vi "Convert RGB to HSV.vi"(11 "Color Box":u32(colorbox)=16777215) -> (1 "V (%)":dbl, 2 "S (%)":dbl, 3 "H (deg)":dbl format="%#_2p")   [LabVIEW 2014, in "HSV Distance Comparison.lvclass"]
doc: "This VI will convert the RGB Color Scale to the HSL Color Scale.\n<b> </b> <b> </b>\n©2017 Q Software Innovations, LLC (QSI)\nwritten by Quentin Alldredge\nproduced in LabVIEW 2015\n\nsupport@qsoftwareinnovations.com\nwww.qsoftwareinnovations.com\n\nAll rights reserved.\n\nRedistribution and use in source and binary forms, with or without modification, are permitted provided that the following conditions are met:\n\n * Redistributions of source code must retain the above copyright notice, this list of conditions and the following disclaimer.\n * Redistributions in binary form must reproduce the above copyright notice, this list of conditions and the following disclaimer in the documentation and/or other materials provided with the distribution.\n * Neither the name of Q Software Innovations, LLC. nor the names of its contributors may be used to endorse or promote products derived from this software without specific prior written permission.\n\nTHIS SOFTWARE IS PROVIDED BY THE COPYRIGHT HOLDERS AND CONTRIBUTORS \"AS IS\" AND ANY EXPRESS OR IMPLIED WARRANTIES, INCLUDING, BUT NOT LIMITED TO, THE IMPLIED WARRANTIES OF MERCHANTABILITY AND FITNESS FOR A PARTICULAR PURPOSE ARE DISCLAIMED. IN NO EVENT SHALL THE COPYRIGHT OWNER OR CONTRIBUTORS BE LIABLE FOR ANY DIRECT, INDIRECT, INCIDENTAL, SPECIAL, EXEMPLARY, OR CONSEQUENTIAL DAMAGES (INCLUDING, BUT NOT LIMITED TO, PROCUREMENT OF SUBSTITUTE GOODS OR SERVICES; LOSS OF USE, DATA, OR PROFITS; OR BUSINESS INTERRUPTION) HOWEVER CAUSED AND ON ANY THEORY OF LIABILITY, WHETHER IN CONTRACT, STRICT LIABILITY, OR TORT (INCLUDING NEGLIGENCE OR OTHERWISE) ARISING IN ANY WAY OUT OF THE USE OF THIS SOFTWARE, EVEN IF ADVISED OF THE POSSIBILITY OF SUCH DAMAGE."
uses:
  HSV Distance Comparison.lvclass
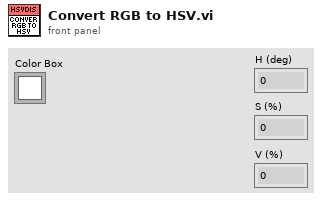
[diagram p1: front panel]
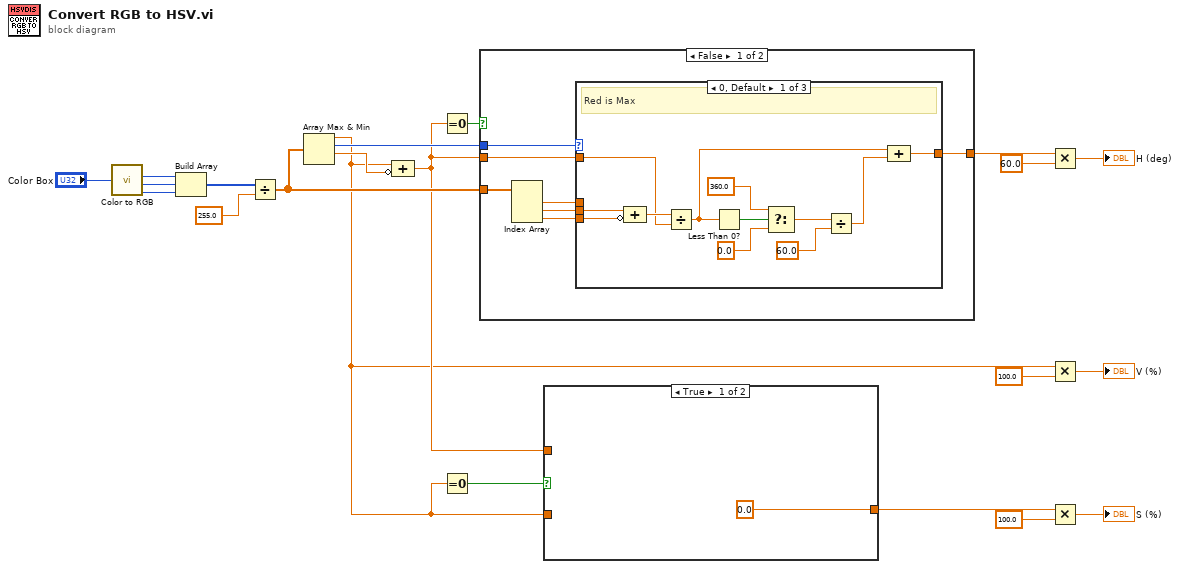
[diagram p0: block diagram]
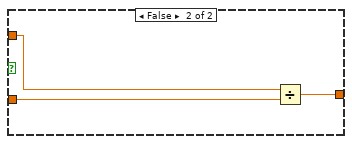
[diagram p2: hidden frame]
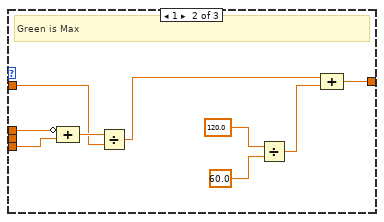
[diagram p3: hidden frame]
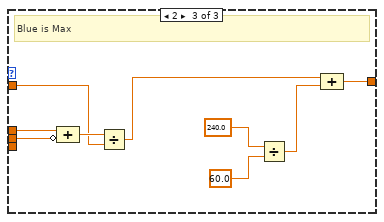
[diagram p4: hidden frame]
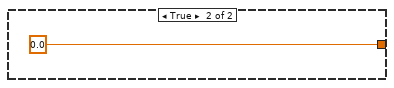
[diagram p5: hidden frame]
diagram:
  n1 = call <vilib>:"Color to RGB.vi"("Color"="Color Box") -> ("R"=w6:u8, "G"=w5:u8, "B"=w4:u8)  [unwired: 1 out]
  n2 = Build Array(w6, w5, w4) -> (w17:u8[])
  n3 = Divide(x=w17, y=255.0 ("x")) -> (x/y=w15:dbl[])
  n4 = Array Max & Min(array=w15) -> (max value=w1:dbl, max index (indices)=w19:i32, min value=w20:dbl)  [unwired: 1 out]
  n5 = Compound Arithmetic op=ADD(w1, invert w20) -> (w2:dbl)
  n6 = Equal To 0?(x=w2) -> (x = 0?=w3:bool)
  n7 = Equal To 0?(x=w1) -> (x = 0?=w18:bool)
  n8 = case shown="False" w3 {
    tunnel: [w27 0.0] -> w13
    tunnel: w19 -> [w28 _]
    tunnel: w15 -> [w26 _]
    tunnel: w2 -> [w22 _]
    frame False {
      n9 = Index Array(array=w26) -> (element #1=w25:dbl, element #2=w24:dbl, element #3=w23:dbl)  [unwired: 3 in]
      n10 = case shown="0, Default" w28 {
        tunnel: w22 -> [w39 w48 w57]
        tunnel: [w31 w44 w53] -> w27
        tunnel: w25 -> [_ w42 w51]
        tunnel: w24 -> [w30 _ w50]
        tunnel: w23 -> [w29 w41 _]
        frame 0, Default {
          # "Red is Max"
          n11 = Compound Arithmetic op=ADD(w30, invert w29) -> (w40:dbl)
          n12 = Divide(x=w40, y=w39) -> (x/y=w33:dbl)
          n13 = Less Than 0?(x=w33) -> (x < 0?=w38:bool)
          n14 = Select(t=360.0 ("x"), s=w38, f=0.0 ("x")) -> (s? t:f=w35:dbl)
          n15 = Divide(x=w35, y=60.0) -> (x/y=w32:dbl)
          n16 = Compound Arithmetic op=ADD(w33, w32) -> (w31:dbl)
        }
        frame 1 {
          # "Green is Max"
          n17 = Compound Arithmetic op=ADD(invert w42, w41) -> (w49:dbl)
          n18 = Divide(x=w49, y=w48) -> (x/y=w46:dbl)
          n19 = Divide(x=120.0, y=60.0) -> (x/y=w45:dbl)
          n20 = Compound Arithmetic op=ADD(w46, w45) -> (w44:dbl)
        }
        frame 2 {
          # "Blue is Max"
          n21 = Compound Arithmetic op=ADD(w51, invert w50) -> (w58:dbl)
          n22 = Divide(x=w58, y=w57) -> (x/y=w55:dbl)
          n23 = Divide(x=240.0, y=60.0) -> (x/y=w54:dbl)
          n24 = Compound Arithmetic op=ADD(w55, w54) -> (w53:dbl)
        }
      }
    }
    frame True {
    }
  }
  n25 = case shown="True" w18 {
    tunnel: [0.0 ("y") w62] -> w8
    tunnel: w1 -> [_ w63]
    tunnel: w2 -> [_ w61]
    frame True {
    }
    frame False {
      n26 = Divide(x=w61, y=w63) -> (x/y=w62:dbl)
    }
  }
  n27 = Multiply(x=w13, y=60.0) -> (x*y=→"H (deg)":dbl)
  n28 = Multiply(x=w1, y=100.0) -> (x*y=→"V (%)":dbl)
  n29 = Multiply(x=w8, y=100.0) -> (x*y=→"S (%)":dbl)
